vi "New Boolean Text Binding.vi"(7 "Format String":string, 10 "Bool Refnum":refnum<vi>) -> (0 "error out":errorcluster, 3 "BooleanTextBinding Out":refnum<class "BooleanTextBinding.lvclass">)   [LabVIEW 2015, in "Transport.lvlib" / "BooleanTextBinding.lvclass"]
doc: "<License>\nCopyright © 2017 Composed Systems, LLC | All rights reserved\nwww.composed.io\n\nAuthor: Ethan Stern <ethan.stern@composed.io>\n\nThis software is provided \"AS IS\" WITHOUT WARRANTIES, either express or implied, AND IS FOR EDUCATIONAL PURPOSES ONLY.\n</License>"
uses:
  BooleanTextBinding.lvclass
  BooleanTextBinding.lvclass/BooleanTextBinding.ctl
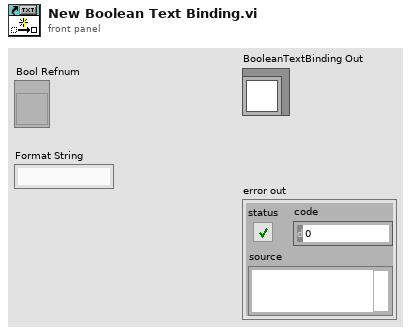
[diagram p1: front panel]
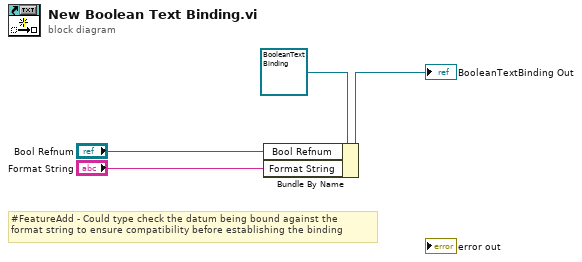
[diagram p0: block diagram]
diagram:
  # "#FeatureAdd - Could type check the datum being bound against the\nformat string to ensure compatibility before establishing the binding"
  n1 = Bundle By Name(cluster=refnum<class "BooleanTextBinding.lvclass"> refnum ("TerminalBinding in"), "Bool Refnum"="Bool Refnum", "Format String"="Format String") -> (→"BooleanTextBinding Out":refnum<class "BooleanTextBinding.lvclass">)
